vi "DrawFormattedMultilineString.vi"(0 "reference":refnum<class "Graphics.lvclass">, 1 "text":string, 2 "bounds":T1 {"height" format="%.2f"; "width" format="%.2f"; "y" format="%.2f"; "x" format="%.2f"}, 3 "fontType":T5, 4 "font":T4, 5 "error in (no error)":errorcluster, 7 "alignment(left, top)":T3, 9 "Justification":T2, 11 "GAP":i32) -> (14 "reference out":refnum<class "Graphics.lvclass">, 19 "error out":errorcluster)   [LabVIEW 2014, in "Graphics.lvclass"]
uses:
  <resource>/Framework/Providers/Open_GDS/UML/Graphics_class/Graphics.lvclass
  <resource>/Framework/Providers/Open_GDS/UML/Graphics_class/LvFontType.ctl
  <resource>/Framework/Providers/Open_GDS/UML/Graphics_class/FontType.ctl
  <resource>/Framework/Providers/Open_GDS/UML/MultiLineString_class/JustificationType.ctl
  <resource>/Framework/Providers/Open_GDS/UML/General/Rectangle/Rectangle Rectangle2D.ctl
  <resource>/Framework/Providers/Open_GDS/UML/MultiLineString_class/MultiLineString.lvclass
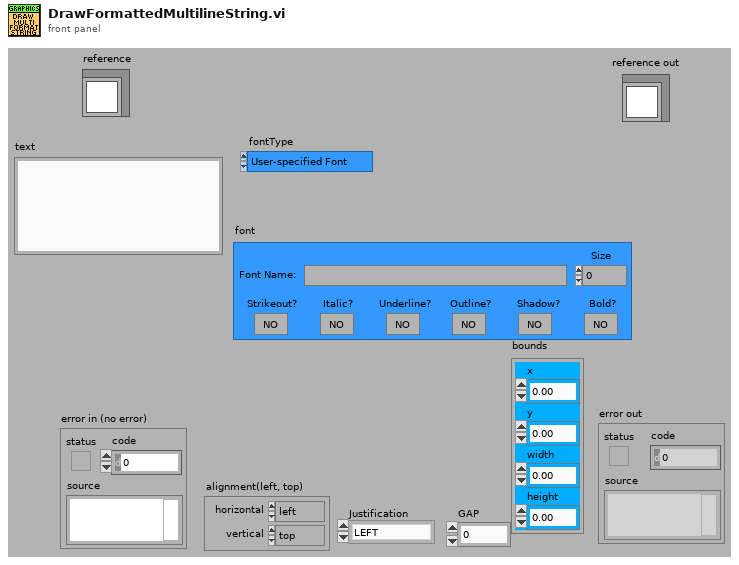
[diagram p1: front panel]
types:
  T1 = typedef "Rectangle Rectangle2D.ctl" = cluster{"x":dbl, "y":dbl, "width":dbl, "height":dbl}
  T2 = typedef "MultiLineString.lvclass/JustificationType.ctl" = enum16{"LEFT", "CENTER", "RIGHT"}
  T3 = cluster{"horizontal":enum16{"left", "center", "right"}, "vertical":enum16{"top", "center", "bottom"}}
  T4 = typedef "Graphics.lvclass/FontType.ctl" = cluster{"Font Name:":string, "Size":i16, "Strikeout?":bool, "Italic?":bool, "Underline?":bool, "Outline?":bool, "Shadow?":bool, "Bold?":bool}
  T5 = typedef "Graphics.lvclass/LvFontType.ctl" = enum16{"User-specified Font", "Application Font", "System Font", "Dialog Font"}
  T6 = typedef "Graphics.lvclass/ObjectAttributes.ctl" = cluster{"drawColor":u32, "backgroundColor":u32, "font":T4, "fontType":T5, "picture":picture, "stroke":T7, "scaleX":dbl, "scaleY":dbl, "screenRef":refnum<vi>, "offsetX":dbl, "offsetY":dbl}
  T7 = typedef "Graphics.lvclass/StrokeType.ctl" = enum16{"USE_DEFAULT", "SOLID", "DOTTED"}
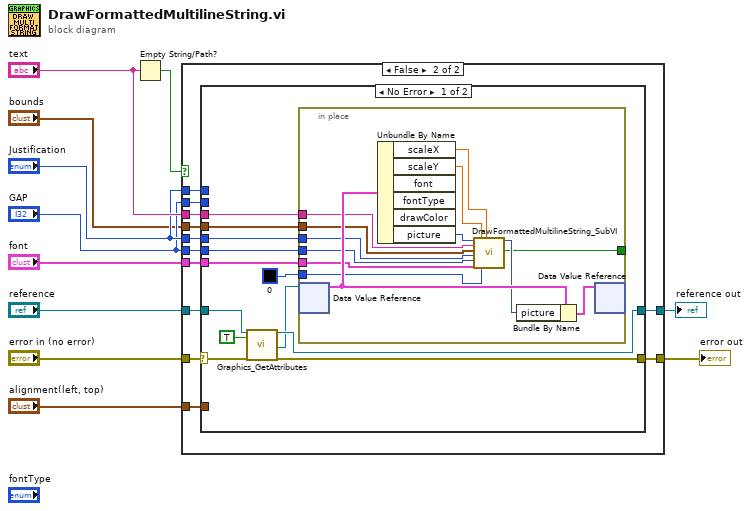
[diagram p0: block diagram]
diagram:
  n1 = Empty String/Path?(string/path="text") -> (empty?=w4:bool)
  n2 = case shown="False" w4 {
    tunnel: "error in (no error)" -> [w12 w25]
    tunnel: "reference" -> [w13 w24]
    tunnel: [w12 w23] -> w9
    tunnel: [w13 w22] -> w8
    tunnel: "font" -> [_ w21]
    tunnel: "alignment(left, top)" -> [_ w20]
    tunnel: "text" -> [_ w19]
    tunnel: "Justification" -> [_ w18]
    tunnel: "GAP" -> [_ w17]
    tunnel: "Justification" -> [_ w16]
    tunnel: "GAP" -> [_ w15]
    tunnel: "bounds" -> [_ w14]
    frame True {
    }
    frame False {
      n3 = case shown="No Error" w25 {
        selector: w25 -> [w37 w51]
        tunnel: w24 -> [w36 w52]
        tunnel: [w35 w51] -> w23
        tunnel: [w34 w52] -> w22
        tunnel: w19 -> [w31 _]
        tunnel: w21 -> [w27 _]
        tunnel: w20 -> [_ _]
        tunnel: w18 -> [_ _]
        tunnel: w17 -> [_ _]
        tunnel: w16 -> [w29 _]
        tunnel: w15 -> [w28 _]
        tunnel: w14 -> [w30 _]
        frame No Error {
          n4 = call <resource>:"Graphics_GetAttributes.vi"("reference in"=w36, "OnlyGetDvrReference(False)"=TRUE, "error in (no error)"=w37) -> ("reference out"=w34:refnum<class "Graphics.lvclass">, "DataRef"=w32:refnum<data-value>, "error out"=w35:errorcluster)  [unwired: 13 in, 1 out]
          n5 = in-place {
            in-place-border: w31 -> [w44]
            in-place-border: w30 -> [w43]
            in-place-border: w29 -> [w42]
            in-place-border: w28 -> [w41]
            in-place-border: w27 -> [w40]
            in-place-border: u32 0 ("Color") -> [w39]
            in-place-border: [w38] -> _
            n6 = in-place-dvr #1(w32) -> (w50:T6)  [unwired: 1 out]
            n7 = Unbundle By Name(w50) -> ("scaleX"=w47:dbl, "scaleY"=w46:dbl, "picture"=w45:picture)  [unwired: 3 out]
            n8 = call <resource>:"DrawFormattedMultilineString_SubVI.vi"("PictureIn"=w45, "FormattedMultiLineStringIn"=w44, "TextRectangle"=w43, "Justification"=w42, "GAP"=w41, "Font"=w40, "scaleY"=w46, "Color"=w39, "scaleX"=w47) -> ("PictureOut"=w49:picture, "NoChange"=w38:bool)  [unwired: 9 in]
            n9 = Bundle By Name(cluster=w50, "picture"=w49) -> (w48:T6)
            n10 = in-place-dvr #1(w48) -> ()  [unwired: 2 out]
          }
        }
        frame Error {
        }
      }
    }
  }
  "reference out" <- w8
  "error out" <- w9
